vi "Robot Communication Loop.vi"() -> ()   [LabVIEW 2015]
uses:
  PWM_Output_TypeDef.ctl
  LED_Output_TypeDef.ctl
  <vilib>/Rock Robotics/Network Tables/NT Read Raw.vi
  <vilib>/Rock Robotics/Network Tables/NT Write Raw.vi
panel:
  out "error out":errorcluster
  in  "error in (no error)":errorcluster
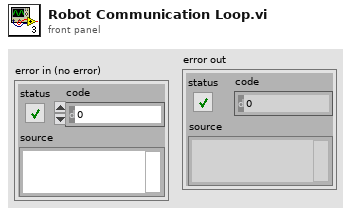
[diagram p1: front panel]
types:
  T1 = typedef "LED_Output_TypeDef.ctl" = cluster{"LED 0":bool, "LED 1":bool, "LED 2":bool, "LED 3":bool, "LED 4":bool, "LED 5":bool, "LED 6":bool, "LED 7":bool, "LED 8":bool, "LED 9":bool, "LED 10":bool, "LED 11":bool, "LED 12":bool, "LED 13":bool, "LED 14":bool, "LED 15":bool}
  T2 = typedef "PWM_Output_TypeDef.ctl" = cluster{"PWM 0":u8, "PWM 1":u8, "PWM 2":u8, "PWM 3":u8, "PWM 4":u8, "PWM 5":u8, "PWM 6":u8, "PWM 7":u8, "PWM 8":u8, "PWM 9":u8, "PWM 10":u8}
  T3 = typedef "Analog_Input_TypeDef.ctl" = cluster{"ANA 0":u8, "ANA 1":u8, "ANA 2":u8, "ANA 3":u8, "ANA 4":u8, "ANA 5":u8, "ANA 6":u8, "ANA 7":u8, "ANA 8":u8, "ANA 9":u8, "ANA 10":u8, "ANA 11":u8, "ANA 12":u8, "ANA 13":u8, "ANA 14":u8, "ANA 15":u8}
  T4 = typedef "Switch_Input_TypeDef.ctl" = cluster{"SW 0":bool, "SW 1":bool, "SW 2":bool, "SW 3":bool, "SW 4":bool, "SW 5":bool, "SW 6":bool, "SW 7":bool, "SW 8":bool, "SW 9":bool, "SW 10":bool, "SW 11":bool, "SW 12":bool, "SW 13":bool, "SW 14":bool, "SW 15":bool}
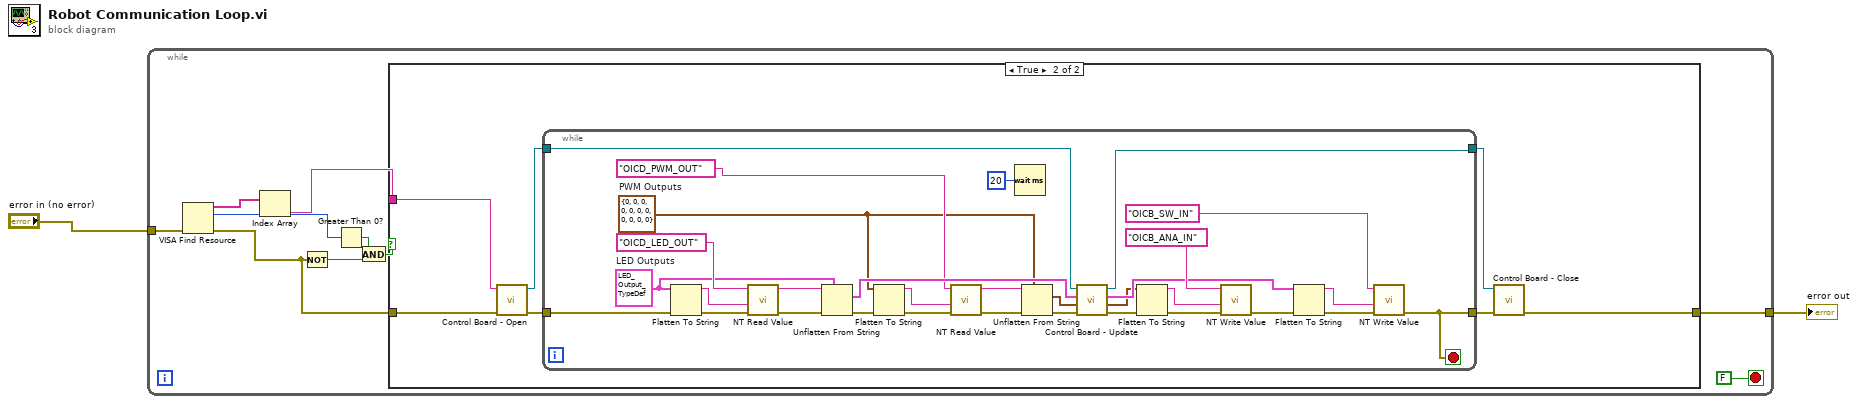
[diagram p0: block diagram]
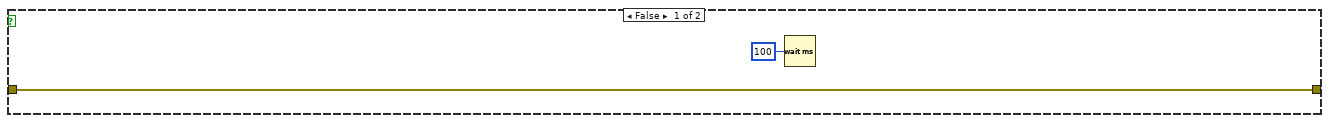
[diagram p2: hidden frame]
diagram:
  n1 = while {
    tunnel: "error in (no error)" -> [w5]
    tunnel: [w3] -> w1
    stop <- FALSE stop-if-true
    n2 = VISA Find Resource(8:w5) -> (0:w4:errorcluster, 2:w12:u32, 3:w11:string[])  [unwired: 2 in]
    n3 = Index Array(array=w11) -> (element=w10:string)  [unwired: 1 in]
    n4 = Not(x=w4) -> (.not. x?=w6:bool)
    n5 = Greater Than 0?(x=w12) -> (x > 0?=w8:bool)
    n6 = And(x=w8, y=w6) -> (x .and. y?=w7:bool)
    n7 = case shown="True" w7 {
      tunnel: w10 -> [_ w17]
      tunnel: w4 -> [w13 w16]
      tunnel: [w13 w15] -> w3
      frame False {
        n8 = Wait (ms)(milliseconds to wait=u32 100) -> ()  [unwired: 1 out]
      }
      frame True {
        n9 = call "Control Board - Open.vi"("error in (no error)"=w16, "VISA Refnum in"=w17) -> ("error out"=w18:errorcluster, "VISA Refnum out"=w21:refnum<visa-resource-name>)  [unwired: 8 in]
        n10 = while {
          tunnel: w21 -> [w52]
          tunnel: [w50] -> w20
          tunnel: [w23] -> w19
          tunnel: w18 -> [w24]
          stop <- w23 stop-if-true
          w31 = T1 {"LED 0"=FALSE, "LED 1"=FALSE, "LED 2"=FALSE, "LED 3"=FALSE, "LED 4"=FALSE, "LED 5"=FALSE, "LED 6"=FALSE, "LED 7"=FALSE, "LED 8"=FALSE, "LED 9"=FALSE, "LED 10"=FALSE, "LED 11"=FALSE, "LED 12"=FALSE, "LED 13"=FALSE, "LED 14"=FALSE, "LED 15"=FALSE}  # LED Outputs
          w29 = T2 {"PWM 0"=0, "PWM 1"=0, "PWM 2"=0, "PWM 3"=0, "PWM 4"=0, "PWM 5"=0, "PWM 6"=0, "PWM 7"=0, "PWM 8"=0, "PWM 9"=0, "PWM 10"=0}  # PWM Outputs
          n11 = Flatten To String(anything=w31, error in (no error)=w24) -> (data string=w30:string, error out=w25:errorcluster)  [unwired: 2 in, 1 out]
          n12 = call-poly <vilib>:"NT Read Value.vi"("error in"=w25, "Default Value"=w30, "Name"="OICD_LED_OUT") -> ("error out"=w38:errorcluster, "Raw"=w40:string)  [unwired: 7 in]
          n13 = Unflatten From String(type=w31, binary string=w40, error in (no error)=w38) -> (value=w42:T1, error out=w26:errorcluster)  [unwired: 2 in, 1 out]
          n14 = Flatten To String(anything=w29, error in (no error)=w26) -> (data string=w28:string, error out=w27:errorcluster)  [unwired: 2 in, 1 out]
          n15 = call-poly <vilib>:"NT Read Value.vi"("error in"=w27, "Default Value"=w28, "Name"="OICD_PWM_OUT") -> ("error out"=w33:errorcluster, "Raw"=w46:string)  [unwired: 7 in]
          n16 = Wait (ms)(milliseconds to wait=u32 20) -> ()  [unwired: 1 out]
          n17 = Unflatten From String(type=w29, binary string=w46, error in (no error)=w33) -> (value=w45:T2, error out=w32:errorcluster)  [unwired: 2 in, 1 out]
          n18 = call "Control Board - Update.vi"("error in (no error)"=w32, "PWM Outputs"=w45, "LED Outputs"=w42, "Control Board VISA Reference In"=w52) -> ("error out"=w35:errorcluster, "Analog Inputs"=w44:T3, "Switch Inputs"=w48:T4, "Control Board VISA Reference Out"=w50:refnum<visa-resource-name>)  [unwired: 4 in]
          n19 = Flatten To String(anything=w44, error in (no error)=w35) -> (data string=w43:string, error out=w37:errorcluster)  [unwired: 2 in, 1 out]
          n20 = call-poly <vilib>:"NT Write Value.vi"("error in"=w37, "Raw"=w43, "Name"="OICB_ANA_IN") -> ("error out"=w34:errorcluster)  [unwired: 8 in]
          n21 = Flatten To String(anything=w48, error in (no error)=w34) -> (data string=w47:string, error out=w36:errorcluster)  [unwired: 2 in, 1 out]
          n22 = call-poly <vilib>:"NT Write Value.vi"("error in"=w36, "Raw"=w47, "Name"="OICB_SW_IN") -> ("error out"=w23:errorcluster)  [unwired: 8 in]
        }
        n23 = call "Control Board - Close.vi"("error in (no error)"=w19, "VISA Refnum in"=w20) -> ("error out"=w15:errorcluster)  [unwired: 9 in]
      }
    }
  }
  "error out" <- w1
